vi "Datum_Turntable_Image.vi"(3 "Mode":T8=enum."Run VI", 5 "Traverse line In":T5={"Start X"=0.0, "Start Y"=nan, "Start Z"=nan, "End X"=nan, "End Y"=nan, "End Z"=nan, "nPoints"=0, "Spacing"=enum."N/A", "Filename"=path "C:/Enflo_Data_Local/2016/EnFlo_Tunnel/Paul_Hayden/Calibrations/Cal_03-2016/Datum_Turntable.xls", "Tunnel Speed"=nan, "Averaging time (mins)"=nan, "Extra Commands"="", "Carrier_1 Q (l/min)"=nan, "Carrier_2 Q (l/min)"=nan, "Trace Gas Concentration (%)"=nan, "Specific Arguments"="Datum_Turntable_Image.vi ", "Comments"="", "Row No"=0, "Row Type Selector"=enum."Run VI Named:", "EstCompl"="12:59  18-03-2016", "Row Duration (mins)"=0.08333333333333333, "nValidPoints"=0, "Meas Setup File"="Trav_Cam_Picture.xls"} {"Carrier_2 Q (l/min)" format="%#.2f"; "Row Duration (mins)" format="%#.1f"; "Row No" min=0; "Trace Gas Concentration (%)" min=0.0 format="%#_4f"; "Carrier_1 Q (l/min)" format="%#.4f"; "Start X" format="%#.2f"; "Start Y" format="%#.2f"; "Start Z" format="%#.2f"; "End X" format="%#.2f"; "End Y" format="%#.2f"; "End Z" format="%#.2f"; "Tunnel Speed" format="%#.2f"; "Averaging time (mins)" min=0.0 format="%#.2f"}) -> (0 "Error Message":string, 1 "Status":T4, 2 "Traverse line Out":T5={"Start X"=0.0, "Start Y"=nan, "Start Z"=nan, "End X"=nan, "End Y"=nan, "End Z"=nan, "nPoints"=0, "Spacing"=enum."N/A", "Filename"=path "C:/Enflo_Data_Local/2016/EnFlo_Tunnel/Paul_Hayden/Calibrations/Cal_03-2016/Datum_Turntable.xls", "Tunnel Speed"=nan, "Averaging time (mins)"=nan, "Extra Commands"="", "Carrier_1 Q (l/min)"=nan, "Carrier_2 Q (l/min)"=nan, "Trace Gas Concentration (%)"=nan, "Specific Arguments"="Datum_Turntable_Image.vi ", "Comments"="", "Row No"=0, "Row Type Selector"=enum."Run VI Named:", "EstCompl"="12:59  18-03-2016", "Row Duration (mins)"=0.08333333333333333, "nValidPoints"=0, "Meas Setup File"="Trav_Cam_Picture.xls"} {"Carrier_2 Q (l/min)" format="%#.2f"; "Row Duration (mins)" format="%#.1f"; "Row No" min=0; "Trace Gas Concentration (%)" min=0.0 format="%#_4f"; "Carrier_1 Q (l/min)" format="%#.4f"; "Start X" format="%#.2f"; "Start Y" format="%#.2f"; "Start Z" format="%#.2f"; "End X" format="%#.2f"; "End Y" format="%#.2f"; "End Z" format="%#.2f"; "Tunnel Speed" format="%#.2f"; "Averaging time (mins)" min=0.0 format="%#.2f"})   [LabVIEW 2021]
uses:
  Gen Trav/Traverse_cluster.ctl
  Gen Trav/Spacing.ctl
  Controls/Multi_run_mode.ctl
  Controls/User_Specific_mode.ctl
  Gen Trav/Multi_Run_Status.ctl
  Utilities/Image acquisition and processing/Feature detection/Typedefs/ROI bounds.ctl
  Utilities/Image acquisition and processing/Feature detection/Typedefs/Theta range.ctl
  Utilities/Image acquisition and processing/Feature detection/Typedefs/Top level controls.ctl
  Camera Server/Camera enum/Camera resolution.ctl
  Gen Trav/Trav_mode.ctl
  Controls/Tunnel_Coordinates.ctl
  Utilities/Image acquisition and processing/Feature detection/Typedefs/Txy range.ctl
panel:
  out "Deg for Relaxing Drive":dbl
  in  "Controls":T1={"Auto ROI (for rot.)"=TRUE, "Apply scaling"=FALSE, "Apply rotation"=TRUE, "Apply Tx"=TRUE, "Apply Ty"=TRUE, "Keep proc. img"=FALSE}
  in  "Theta range (deg)":T2={"theta max (deg)"=180.0, "theta min (deg)"=-180.0}
  in  "ROI to crop (pixels)":T3={"Xmax"=1612, "Ymax"=1300, "Xmin"=660, "Ymin"=226}
  # "X           Y          Z"
  # "Start"
  # "End"
  # "X           Y          Z"
  # "Start"
  # "End"
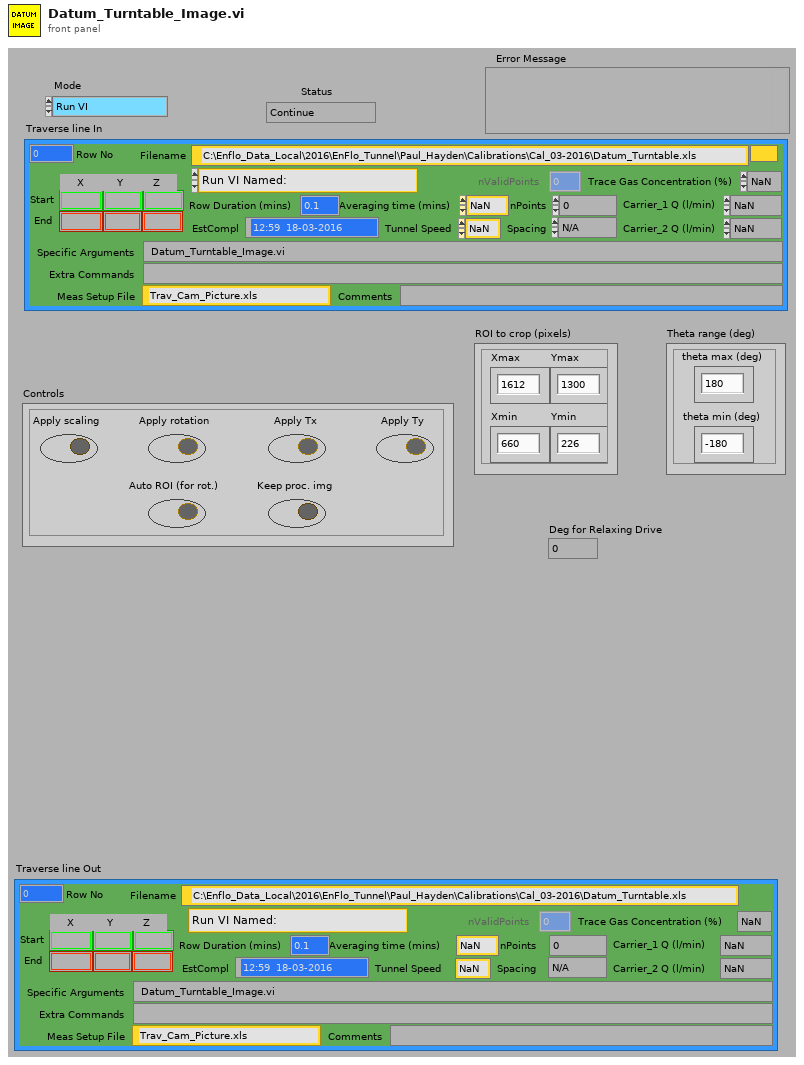
[diagram p1: front panel]
types:
  T1 = typedef "Top level controls.ctl" = cluster{"Auto ROI (for rot.)":bool, "Apply scaling":bool, "Apply rotation":bool, "Apply Tx":bool, "Apply Ty":bool, "Keep proc. img":bool}
  T2 = typedef "Theta range.ctl" = cluster{"theta max (deg)":dbl, "theta min (deg)":dbl}
  T3 = typedef "ROI bounds.ctl" = cluster{"Xmax":i32, "Ymax":i32, "Xmin":i32, "Ymin":i32}
  T4 = typedef "Multi_Run_Status.ctl" = enum16{"Continue", "Continue with Error", "Jump to Next Point", "Jump to Next Row", "Jump To Fall Back", "Terminate Run"}
  T5 = typedef "Traverse_cluster.ctl" = cluster{"Start X":sgl, "Start Y":sgl, "Start Z":sgl, "End X":sgl, "End Y":sgl, "End Z":sgl, "nPoints":i32, "Spacing":T6, "Filename":path, "Tunnel Speed":dbl, "Averaging time (mins)":dbl, "Extra Commands":string, "Carrier_1 Q (l/min)":dbl, "Carrier_2 Q (l/min)":dbl, "Trace Gas Concentration (%)":dbl, "Specific Arguments":string, "Comments":string, "Row No":i32, "Row Type Selector":T7, "EstCompl":string, "Row Duration (mins)":dbl, "nValidPoints":i32, "Meas Setup File":string}
  T6 = typedef "Spacing.ctl" = enum16{"Linear", "Log", "Gauss", "Specified", "N/A"}
  T7 = typedef "Multi_run_mode.ctl" = enum16{"Move Traverse Only", "Set Tunnel Speed Only", "Set Source Only", "Set Measurement Conditions", "Single Measurement", "Vertical Profile", "Lateral Profile", "Longitudinal Profile", "Multi-Axis Profile", "Explore Volume", "Auto Calibrate", "Meas Fast FID Bkgnd", "Check Beam Power", "Scanning Valve Measurement", "Run VI Named:", "Set ADAM Ch", "Wait (minutes)", "Send Message", "Synchronize With:", "Fall Back to this Row", "Turn Off Row Repeating", "Traverse 3D Volume", "Blank Row", "Jump to Fall Back Row"}
  T8 = typedef "User_Specific_mode.ctl" = enum16{"Check VI only", "Run VI"}
  T9 = typedef "Camera resolution.ctl" = u8
  T10 = typedef "Tunnel_Coordinates.ctl" = enum16{"Work in Tunnel Coordinates", "Work in Model Coordinates"}
  T11 = typedef "Trav_mode.ctl" = enum16{"Move traverse", "Read traverse position", "Teach Position"}
  T12 = typedef "Txy range.ctl" = cluster{"Tx max (pix)":i32, "Tx min (pix)":i32, "Ty max (pix)":i32, "Ty min (pix)":i32}
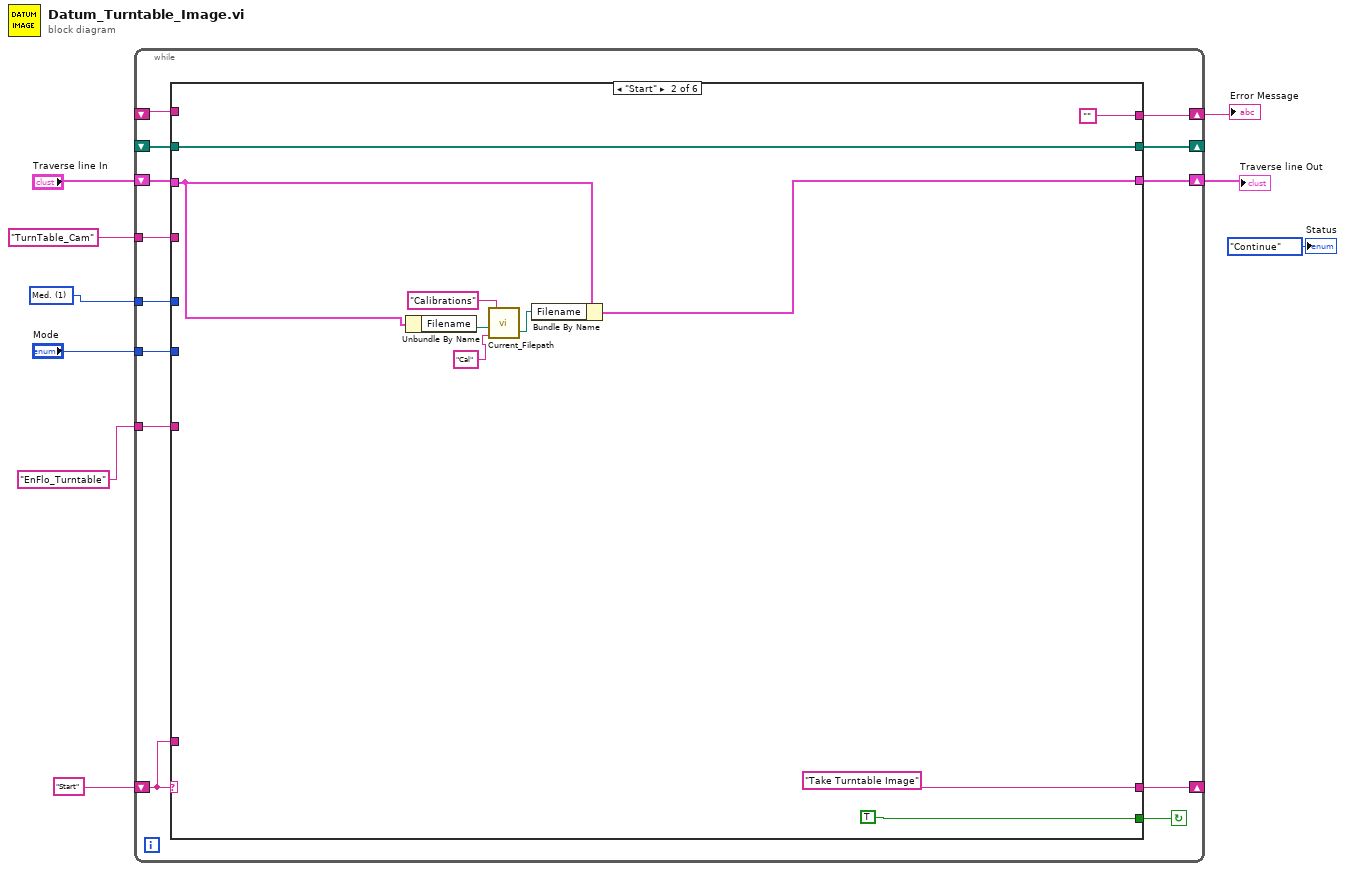
[diagram p0: block diagram]
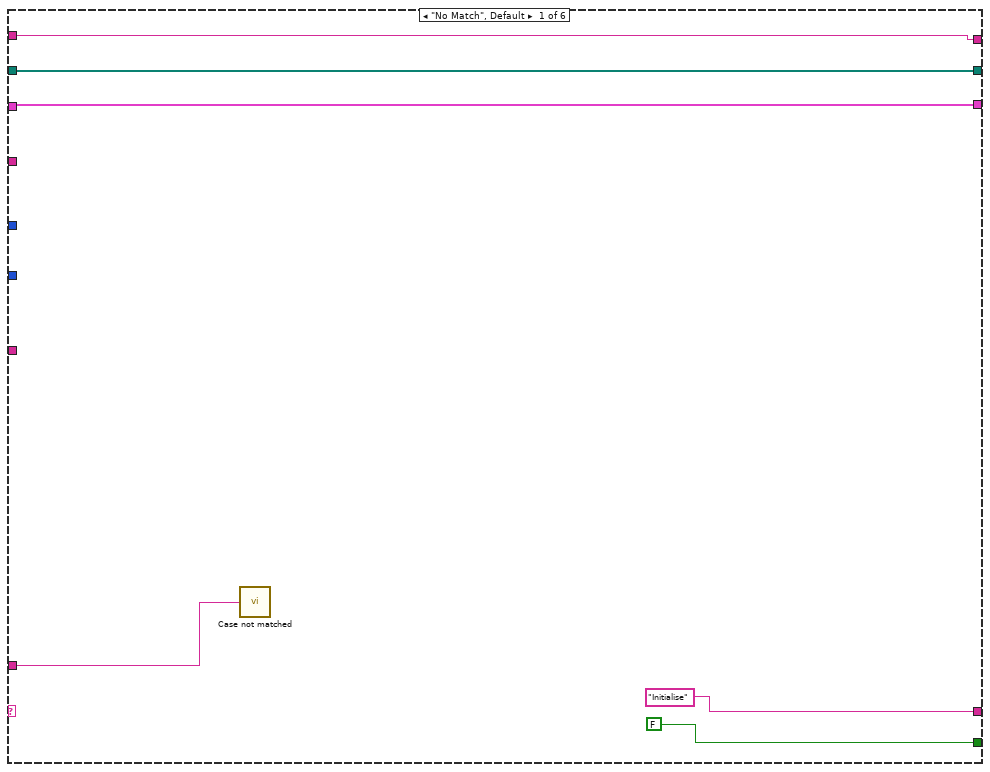
[diagram p2: hidden frame]
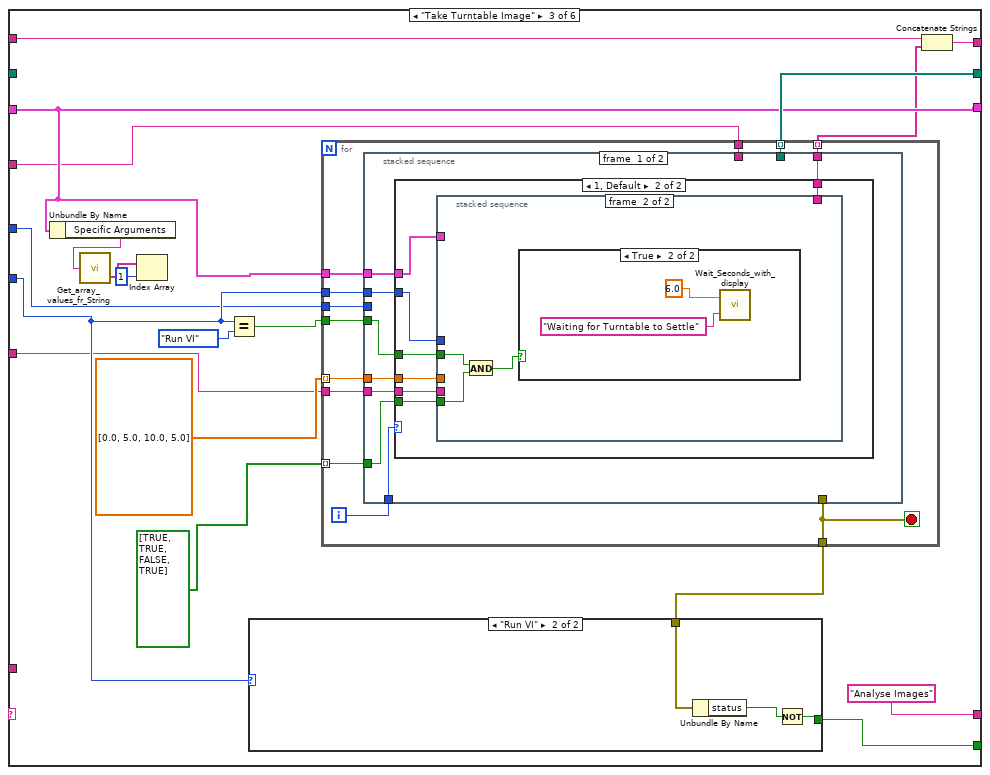
[diagram p3: hidden frame]
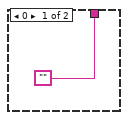
[diagram p4: hidden frame]
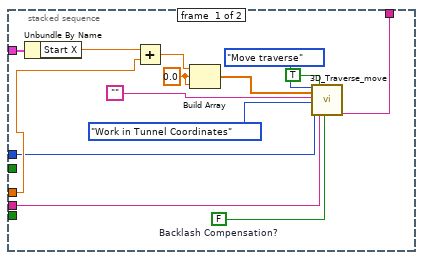
[diagram p5: hidden frame]
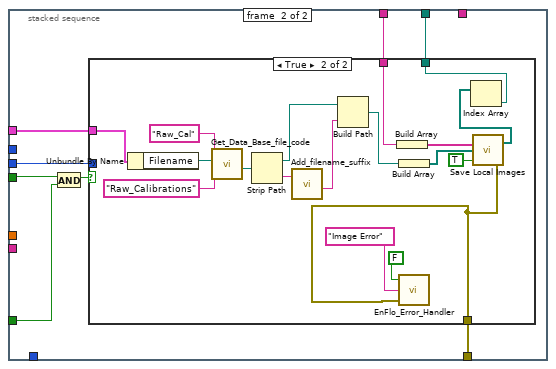
[diagram p7: hidden frame]
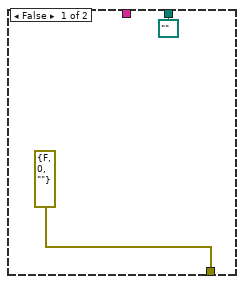
[diagram p8: hidden frame]
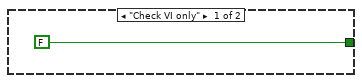
[diagram p9: hidden frame]
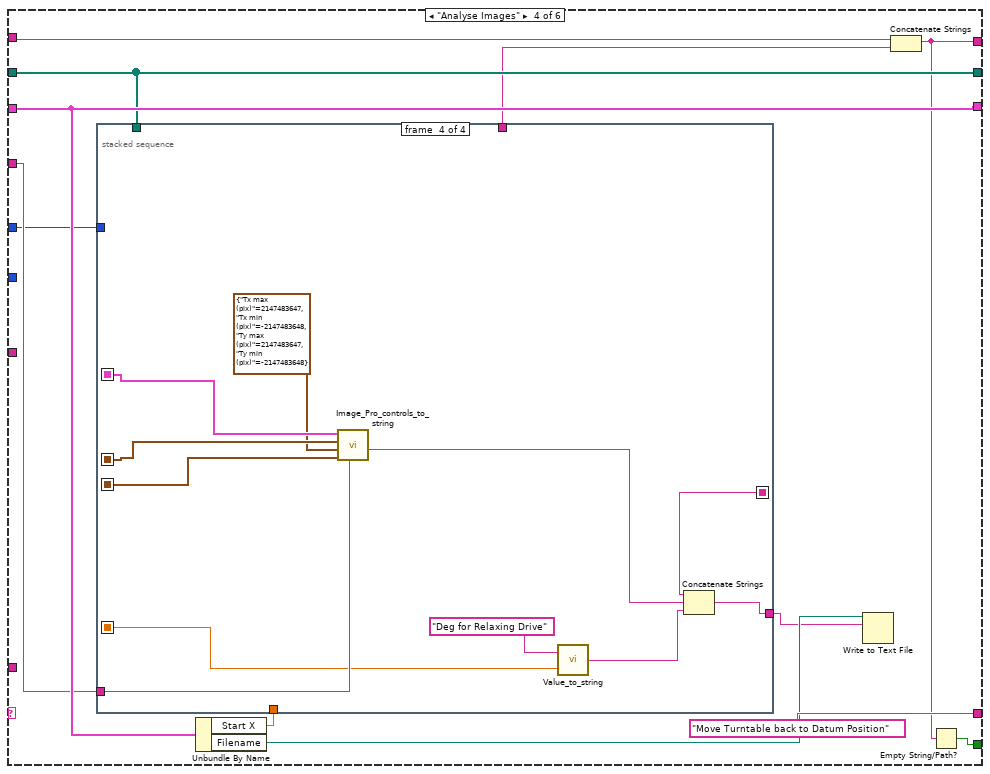
[diagram p10: hidden frame]
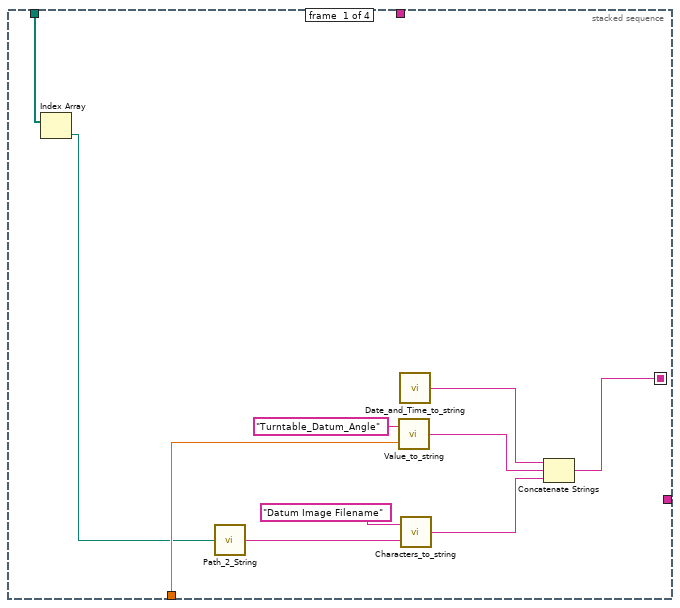
[diagram p11: hidden frame]
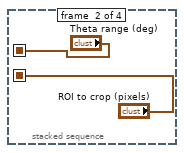
[diagram p12: hidden frame]
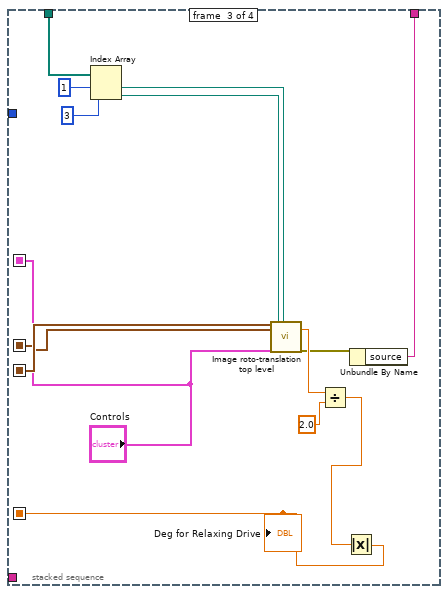
[diagram p13: hidden frame]
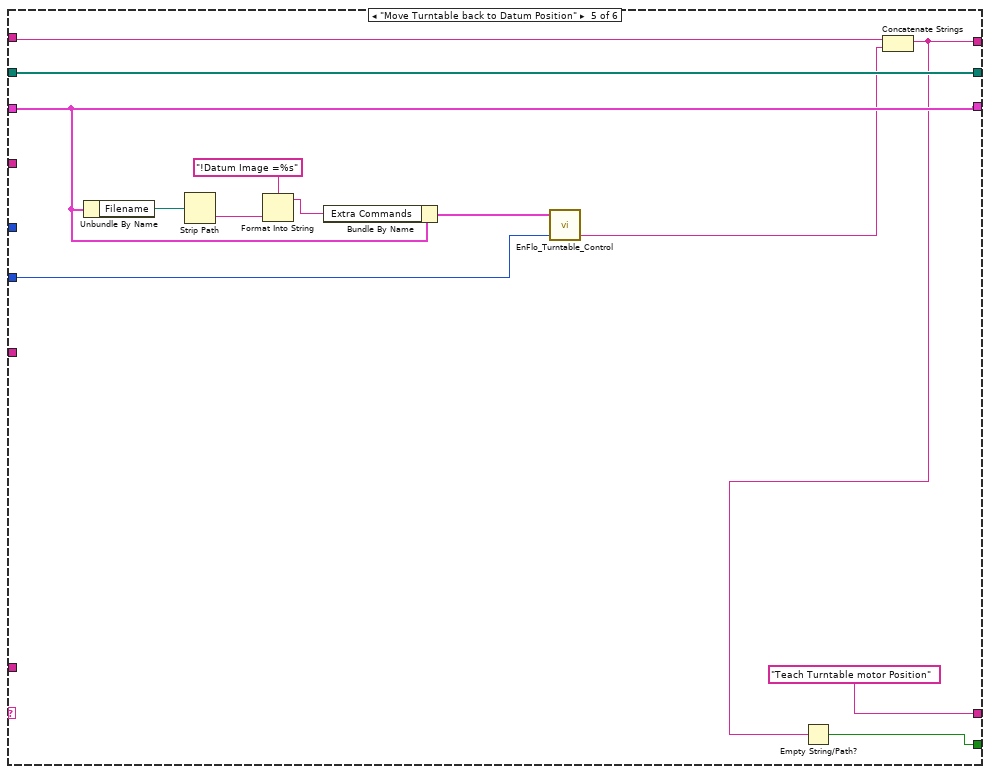
[diagram p14: hidden frame]
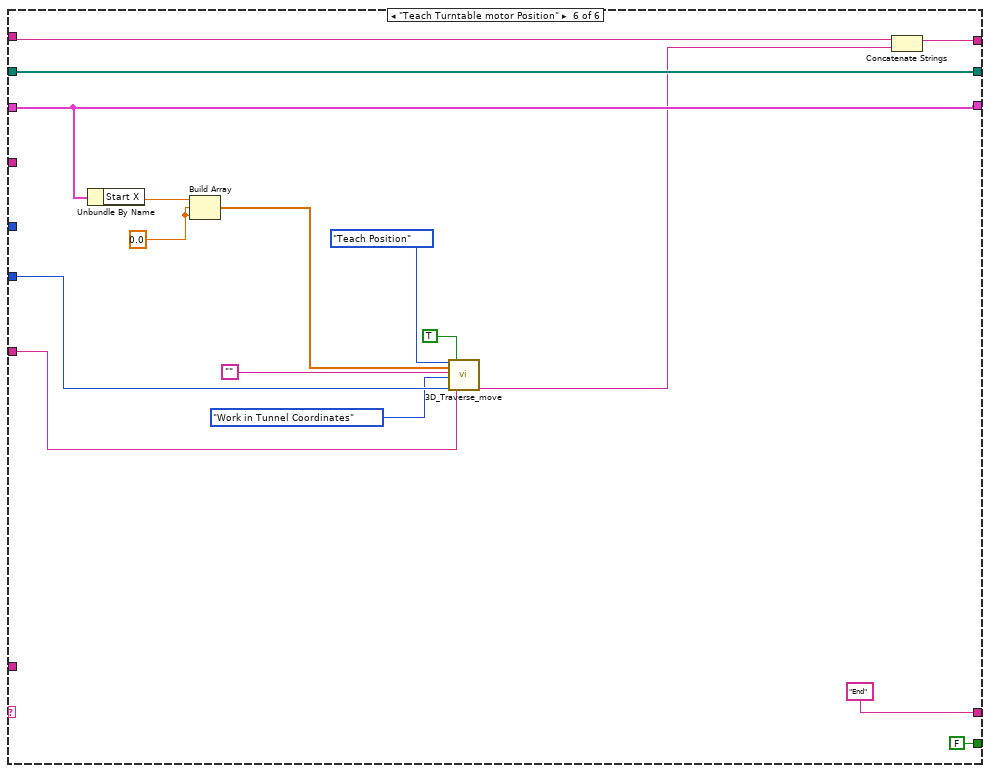
[diagram p15: hidden frame]
diagram:
  w3 = T9 1 items=["Low", "Med.", "High", "Max."] ("Resolution")
  n1 = while {
    shift-left: "Start" -> [w20]
    shift-right: [w21] -> _
    tunnel: "Mode" -> [w19]
    shift-right: [w17] -> w5
    shift-left: "Traverse line In" -> [w18]
    shift-right: [w16] -> _
    shift-left: _ -> [w15]
    tunnel: "TurnTable_Cam" -> [w14]
    shift-right: [w12] -> w4
    shift-left: _ -> [w13]
    tunnel: w3 -> [w11]
    tunnel: "EnFlo_Turntable" -> [w10]
    stop <- w22 continue-if-true
    n2 = case shown="\"Start\"" w20 {
      tunnel: [FALSE TRUE w55 w138 w189 FALSE] -> w22
      tunnel: ["Initialise" "Take Turntable Image" "Analyse Images" "Move Turntable back to Datum Position" "Teach Turntable motor Position" "End"] -> w21
      tunnel: w20 -> [w23 _ _ _ _ _]
      tunnel: w19 -> [_ _ w44 _ w190 w211]
      tunnel: w18 -> [w26 w33 w53 w147 w195 w210]
      tunnel: [w26 w32 w53 w147 w195 w210] -> w17
      tunnel: [w25 w31 w56 w142 w197 w213] -> w16
      tunnel: w15 -> [w25 w31 _ w142 w197 w213]
      tunnel: w14 -> [_ _ w49 w144 _ _]
      tunnel: w13 -> [w24 _ w42 w140 w188 w206]
      tunnel: [w24 "" w41 w139 w186 w204] -> w12
      tunnel: w11 -> [_ _ w40 w137 _ _]
      tunnel: w10 -> [_ _ w39 _ _ w200]
      frame "No Match", Default {
        n3 = call "Case not matched.vi"("Case Name not Matched"=w23) -> ()
      }
      frame "Start" {
        n4 = Unbundle By Name(w33) -> ("Filename"=w35:path)
        n5 = call "Current_Filepath.vi"("Short_Name"="Cal" ("Data Type"), "Filename in"=w35, "Data Type"="Calibrations") -> ("Filename Out"=w30:path)  [unwired: 1 in, 1 out]
        n6 = Bundle By Name(cluster=w33, "Filename"=w30) -> (w32:T5)
      }
      frame "Take Turntable Image" {
        n7 = Unbundle By Name(w53) -> ("Specific Arguments"=w52:string)
        n8 = call "Get_array_values_fr_String.vi"("String Value"=w52) -> ("String array"=w51:string[])  [unwired: 1 out]
        n9 = Index Array(array=w51, index=1) -> ()  [unwired: 1 out]
        n10 = Equal?(x=w44, y=User_Specific_mode."Run VI" ("Mode")) -> (x = y?=w46:bool)
        n11 = for {
          tunnel: [w69] -> w56 mode=indexing
          tunnel: w46 -> [w68]
          tunnel: [w58] -> w54
          tunnel: w53 -> [w67]
          tunnel: w49 -> [w66]
          tunnel: sgl[] [0.0, 5.0, 10.0, 5.0] ("Array") -> [w65] mode=indexing
          tunnel: bool[] [TRUE, TRUE, FALSE, TRUE] ("Array") -> [w63] mode=indexing
          tunnel: w44 -> [w62]
          tunnel: [w61] -> w43 mode=indexing
          tunnel: w40 -> [w60]
          tunnel: w39 -> [w59]
          i -> [w64]
          stop <- w58 stop-if-true
          n12 = stacked-sequence {
            tunnel: [_ w112] -> w69
            tunnel: w68 -> [w74 w108]
            tunnel: [_ w111] -> w58
            tunnel: w67 -> [w77 w110]
            tunnel: w66 -> [_ w109]
            tunnel: w65 -> [w76 _]
            tunnel: w64 -> [w75 _]
            tunnel: w63 -> [w70 w106]
            tunnel: w62 -> [w73 _]
            tunnel: [w72 _] -> w61
            tunnel: w60 -> [_ w105]
            tunnel: w59 -> [w71 _]
            frame #0 {
              n13 = case shown="1, Default" w75 {
                tunnel: w77 -> [_ w85]
                tunnel: w76 -> [_ w84]
                tunnel: w74 -> [_ w81]
                tunnel: w73 -> [_ w83]
                tunnel: ["" w82] -> w72
                tunnel: w71 -> [_ w80]
                tunnel: w70 -> [_ w79]
                frame 0 {
                }
                frame 1, Default {
                  n14 = stacked-sequence {
                    tunnel: w85 -> [w99 _]
                    tunnel: w84 -> [w98 _]
                    tunnel: w83 -> [w89 _]
                    tunnel: [w92 _] -> w82
                    tunnel: w81 -> [_ w102]
                    tunnel: w80 -> [w87 _]
                    tunnel: w79 -> [_ w100]
                    frame #0 {
                      w91 = FALSE  # Backlash Compensation?
                      w95 = sgl 0.0 ("element")
                      n15 = Unbundle By Name(w99) -> ("Start X"=w97:sgl)
                      n16 = Add(x=w97, y=w98) -> (x+y=w96:sgl)
                      n17 = Build Array(w96, w95, w95) -> (w94:sgl[])
                      n18 = call "3D_Traverse_move.vi"("Mode"=Trav_mode."Move traverse", "Position"=w94, "Extra command String"="", "Work in Tunnel Coordinates"=Tunnel_Coordinates."Work in Tunnel Coordinates", "Simulate/Run"=w89, "Route Checking?"=TRUE, "Traverse name"=w87, "Backlash Compensation?"=w91) -> ("Error String"=w92:string)  [unwired: 8 in, 3 out]
                    }
                    frame #1 {
                      n19 = And(x=w102, y=w100) -> (x .and. y?=w101:bool)
                      n20 = case shown="True" w101 {
                        frame False {
                        }
                        frame True {
                          n21 = call "Wait_Seconds_with_display.vi"("Message"="Waiting for Turntable to Settle", "Seconds to wait"=6.0) -> ()  [unwired: 1 in, 1 out]
                        }
                      }
                    }
                  }
                }
              }
            }
            frame #1 {
              n22 = And(x=w108, y=w106) -> (x .and. y?=w107:bool)
              n23 = case shown="True" w107 {
                tunnel: w110 -> [_ w132]
                tunnel: [path "" ("stripped path") w115] -> w112
                tunnel: [errorcluster {"status"=FALSE, "code"=0, "source"=""} ("Error Out") w118] -> w111
                tunnel: w109 -> [_ w124]
                tunnel: w105 -> [_ _]
                frame False {
                }
                frame True {
                  n24 = Unbundle By Name(w132) -> ("Filename"=w128:path)
                  n25 = call "Get_Data_Base_file_code.vi"("Data Type"="Raw_Calibrations", "Results Filename"=w128, "Short_Name"="Raw_Cal" ("Data Type")) -> ("Raw Data File Name"=w127:path)  [unwired: 1 in, 3 out]
                  n26 = Strip Path(path=w127) -> (stripped path=w121:path, name=w129:string)
                  n27 = call "Add_filename_suffix.vi"("Filename"=w129) -> ("Base name"=w120:string)  [unwired: 1 in, 3 out]
                  n28 = Build Path(base path=w121, name or relative path=w120) -> (appended path=w117:path)
                  n29 = Build Array(w124) -> (w123:string[])
                  n30 = Build Array(w117) -> (w122:path[])
                  n31 = call "Save Local Images.vi"("Save Images"=TRUE, "Image Pathnames"=w122, "Camera Names"=w123) -> ("error out"=w118:errorcluster, "Filenames out"=w116:path[])
                  n32 = call "EnFlo_Error_Handler.vi"("error in (no error)"=w118, "Error Type"="Image Error", "Dialog Box (F)"=FALSE ("Dialog Box (T)")) -> ()  [unwired: 1 in, 2 out]
                  n33 = Index Array(array=w116) -> (element=w115:path)  [unwired: 1 in]
                }
              }
            }
          }
        }
        n34 = case shown="\"Run VI\"" w44 {
          tunnel: [FALSE w135] -> w55
          tunnel: w54 -> [_ w136]
          frame "Check VI only" {
          }
          frame "Run VI" {
            n35 = Unbundle By Name(w136) -> ("status"=w134:bool)
            n36 = Not(x=w134) -> (.not. x?=w135:bool)
          }
        }
        n37 = Concatenate Strings(w42, w43) -> (w41:string)
      }
      frame "Analyse Images" {
        n38 = Unbundle By Name(w147) -> ("Start X"=w143:sgl, "Filename"=w146:path)
        n39 = stacked-sequence {
          seq-local: [w153 _ _ _] -> [_ _ _ w178]
          seq-local: [_ "Theta range (deg)" _ _] -> [_ _ w168 w183]
          seq-local: [_ "ROI to crop (pixels)" _ _] -> [_ _ w169 w182]
          seq-local: [_ _ "Controls" _] -> [_ _ _ w184]
          seq-local: [_ _ w163 _] -> [_ _ _ w179]
          tunnel: [_ _ _ w175] -> w145
          tunnel: w144 -> [_ _ _ w185]
          tunnel: w143 -> [w151 _ _ _]
          tunnel: w142 -> [w150 _ w174 _]
          tunnel: [_ _ w161 _] -> w141
          tunnel: w137 -> [_ _ _ _]
          frame #0 {
            n40 = Index Array(array=w150) -> (element=w149:path)  [unwired: 1 in]
            n41 = call "Path_2_String.vi"("Real Path"=w149) -> ("Path String"=w157:string)
            n42 = call "Value_to_string.vi"("Value"=w151, "Label for value"="Turntable_Datum_Angle") -> ("Output string"=w155:string)  [unwired: 1 in]
            n43 = call "Date_and_Time_to_string.vi"() -> ("Date and time (spreadsheet)"=w154:string)  [unwired: 4 in, 1 out]
            n44 = call "Characters_to_string.vi"("Characters to write"=w157, "Label for characters"="Datum Image Filename") -> ("Output string"=w152:string)  [unwired: 1 in]
            n45 = Concatenate Strings(w154, w155, w152) -> (w153:string)
          }
          frame #1 {
          }
          frame #2 {
            n46 = Index Array(array=w174, index #1=1 ("index"), index #2=3 ("index")) -> (element #1=w170:path, element #2=w171:path)
            n47 = call "Image roto-translation top level.vi"("ROI to crop (pixels)"=w169, "Theta range (deg)"=w168, "Controls"="Controls", "Test image file path"=w171, "Reference image file path"=w170) -> ("Rotation (deg)"=w167:dbl, "Error Out"=w162:errorcluster)  [unwired: 7 in, 6 out]
            n48 = Divide(x=w167, y=2.0) -> (x/y=w165:dbl)
            n49 = Absolute Value(x=w165) -> (abs(x)=w163:dbl)
            "Deg for Relaxing Drive" <- w163
            n50 = Unbundle By Name(w162) -> ("source"=w161:string)
          }
          frame #3 {
            n51 = call "Image_Pro_controls_to_string.vi"("Camera"=w185, "ROI to crop (pixels)"=w182, "Txy range (pixels)"=T12 {"Tx max (pix)"=2147483647, "Tx min (pix)"=-2147483648, "Ty max (pix)"=2147483647, "Ty min (pix)"=-2147483648}, "Theta range (deg)"=w183, "Controls"=w184) -> ("Setup String"=w177:string)  [unwired: 6 in]
            n52 = call "Value_to_string.vi"("Value"=w179, "Label for value"="Deg for Relaxing Drive" ("Label for characters")) -> ("Output string"=w176:string)  [unwired: 1 in]
            n53 = Concatenate Strings(w178, w177, w176) -> (w175:string)
          }
        }
        n54 = Write to Text File(file (use dialog)=w146, text=w145) -> ()  [unwired: 2 in, 3 out]
        n55 = Concatenate Strings(w140, w141) -> (w139:string)
        n56 = Empty String/Path?(string/path=w139) -> (empty?=w138:bool)
      }
      frame "Move Turntable back to Datum Position" {
        n57 = Unbundle By Name(w195) -> ("Filename"=w194:path)
        n58 = Strip Path(path=w194) -> (name=w193:string)  [unwired: 1 out]
        n59 = Format Into String(format string="!Datum Image =%s", w193) -> (resulting string=w191:string)  [unwired: 2 in, 1 out]
        n60 = Bundle By Name(cluster=w195, "Extra Commands"=w191) -> (w196:T5)
        n61 = call "EnFlo_Turntable_Control.vi"("Mode"=w190, "Traverse line In"=w196) -> ("Error Message"=w187:string)  [unwired: 1 in, 2 out]
        n62 = Concatenate Strings(w188, w187) -> (w186:string)
        n63 = Empty String/Path?(string/path=w186) -> (empty?=w189:bool)
      }
      frame "Teach Turntable motor Position" {
        w208 = sgl 0.0 ("element")
        n64 = Unbundle By Name(w210) -> ("Start X"=w209:sgl)
        n65 = Build Array(w209, w208, w208) -> (w207:sgl[])
        n66 = call "3D_Traverse_move.vi"("Mode"=Trav_mode."Teach Position", "Position"=w207, "Extra command String"="", "Work in Tunnel Coordinates"=Tunnel_Coordinates."Work in Tunnel Coordinates", "Simulate/Run"=w211, "Route Checking?"=TRUE, "Traverse name"=w200) -> ("Error String"=w205:string)  [unwired: 9 in, 3 out]
        n67 = Concatenate Strings(w206, w205) -> (w204:string)
      }
    }
  }
  "Traverse line Out" <- w5
  "Error Message" <- w4
  "Status" <- Multi_Run_Status."Continue" ("Status")
